vi "웹서버 온도 측정.vi"(6 "참조 번호 입력":T1 caption="client handle out", 7 "physical channels":tag caption="물리적 채널", 8 "error in":errorcluster caption="에러 입력", 9 "thermocouple type":i32(ring)=10072 caption="열전쌍 타입" items=["J"=10072, "K"=10073, "N"=10077, "R"=10082, "S"=10085, "T"=10086, "B"=10047, "E"=10055]) -> (0 "F포맷 문자열":string[](array[string]), 1 "error out":errorcluster, 2 "숫자형":i32, 3 "참조 번호 출력":T1 caption="client handle out", 4 "headers 3":string caption="연결확인 메세지 출력", 5 "온도값":string)   [LabVIEW 2019]
uses:
  <vilib>/httpClient/ClientHandle.ctl
  <vilib>/Analysis/baseanly.llb/Mean (DBL).vi
  <vilib>/DAQmx/read.llb/DAQmx Read (Analog 2D DBL NChan NSamp).vi
  <vilib>/DAQmx/create/channels.llb/DAQmx Create Channel (AI-Temperature-Thermocouple).vi
  <vilib>/DAQmx/configure/timing.llb/DAQmx Timing (Sample Clock).vi
  <vilib>/httpClient/PUTBuffer.vi
  <vilib>/DAQmx/miscellaneous.llb/DAQmx Fill In Error Info.vi
  <vilib>/Analysis/NI_AALBase.lvlib
  <vilib>/httpClient/LabVIEWHTTPClient.lvlib
panel:
  out "data":dbl[][](array[numeric]) caption="데이터" format="%0.2f"
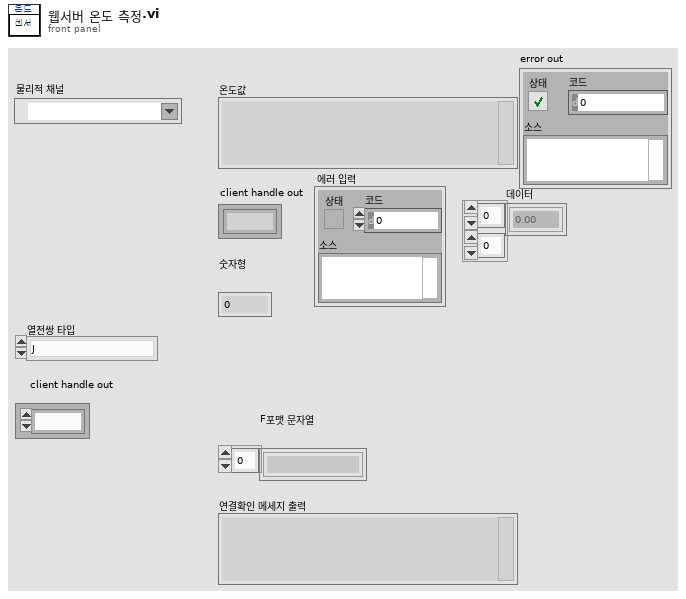
[diagram p1: front panel]
types:
  T1 = typedef "LabVIEWHTTPClient.lvlib/ClientHandle.ctl" = refnum<k1>
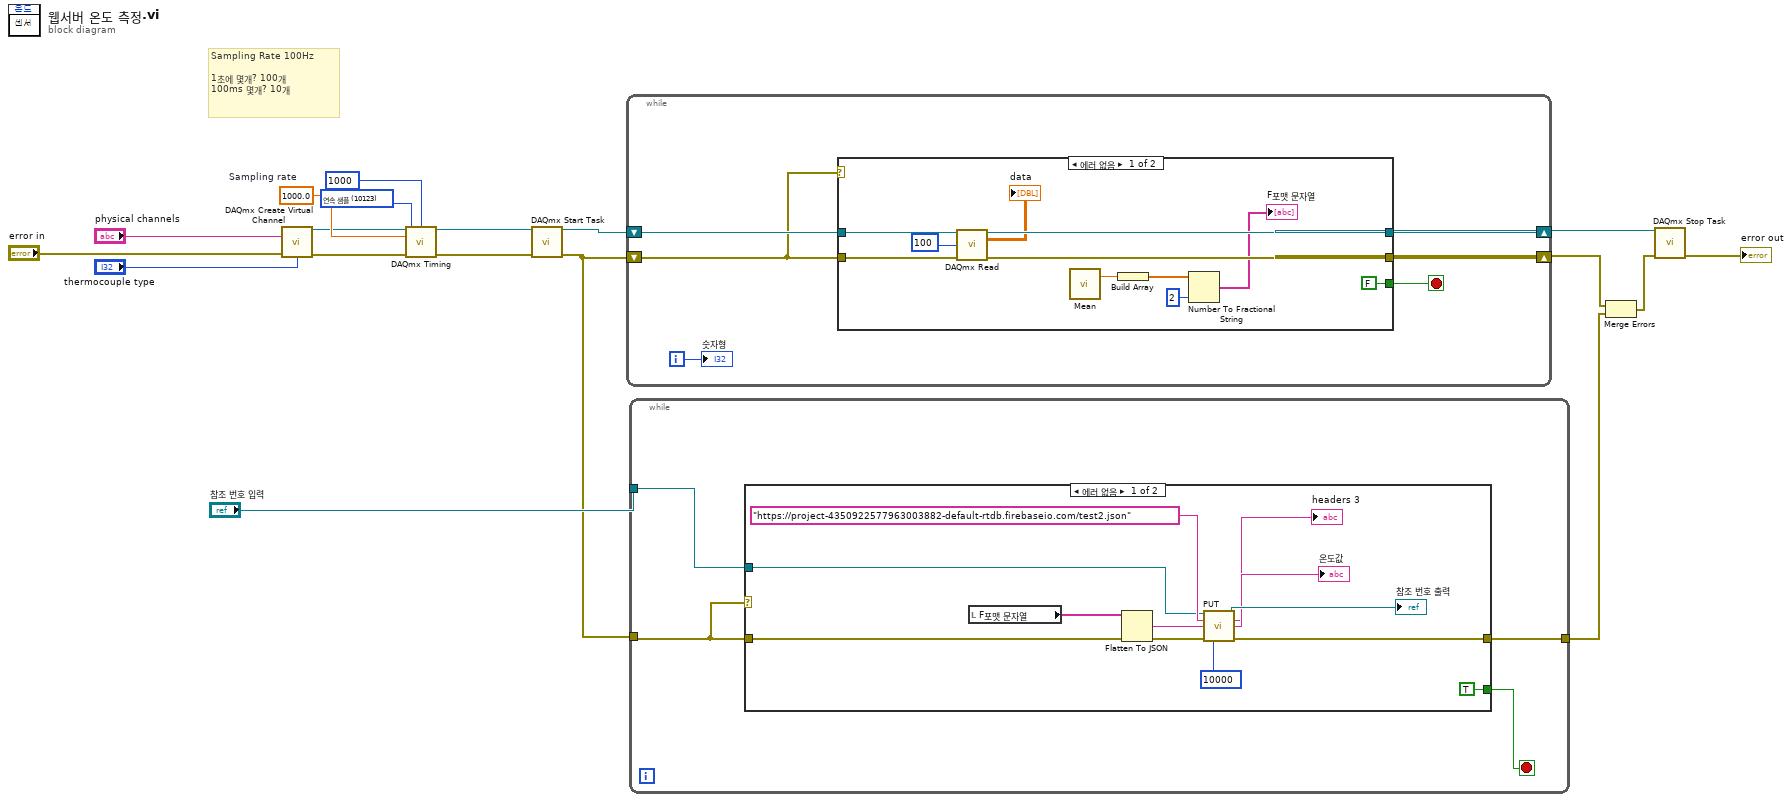
[diagram p0: block diagram]
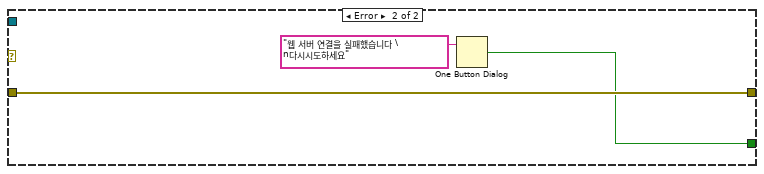
[diagram p2: hidden frame]
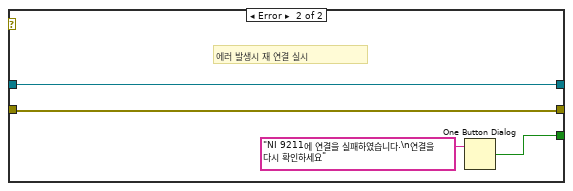
[diagram p3: hidden frame]
diagram:
  w9 = 1000.0  # Sampling rate
  w10 = 10123 items=["유한 샘플"=10178, "연속 샘플"=10123, "하드웨어 타이밍에 의한 단일 포인트"=12522] ("sample mode")
  # "Sampling Rate 100Hz\n\n1초에 몇개? 100개\n100ms 몇개? 10개"
  n1 = call-poly <vilib>:"DAQmx Create Virtual Channel.vi"("physical channels"="physical channels", "error in"="error in", "thermocouple type"="thermocouple type") -> ("task out"=w4:refnum<k21>, "error out"=w6:errorcluster)  [unwired: 11 in]
  n2 = call-poly <vilib>:"DAQmx Timing.vi"("task/channels in"=w4, "sample mode"=w10, "samples per channel"=1000, "rate"=w9, "error in"=w6) -> ("task out"=w5:refnum<k21>, "error out"=w7:errorcluster)  [unwired: 9 in]
  n3 = call <vilib>:"DAQmx Start Task.vi"("task/channels in"=w5, "error in"=w7) -> ("task out"=w12:refnum<k21>, "error out"=w13:errorcluster)  [unwired: 12 in]
  n4 = while {
    shift-right: [w23] -> w11
    shift-left: w12 -> [w24]
    shift-right: [w22] -> w3
    shift-left: w13 -> [w20]
    i -> [w21]
    stop <- w19 stop-if-true
    n5 = case shown="에러 없음" w20 {
      tunnel: w24 -> [w35 w39]
      tunnel: w20 -> [w34 w38]
      tunnel: [w33 w39] -> w23
      tunnel: [w32 w38] -> w22
      tunnel: [FALSE ("true") w36] -> w19
      frame No Error {
        n6 = call-poly <vilib>:"DAQmx Read.vi"("task/channels in"=w35, "number of samples per channel"=100, "error in"=w34) -> ("task out"=w33:refnum<k21>, "data"=→"data":dbl[][], "error out"=w32:errorcluster)  [unwired: 10 in]
        n7 = call-poly <vilib>:"Mean.vi"() -> ("mean"=w28:dbl)  [unwired: 1 in, 1 out]
        n8 = Build Array(w28) -> (w30:dbl[])
        n9 = Number To Fractional String(number=w30, precision (6)=i16 2 ("정밀도(6)")) -> (F-format string=→"F포맷 문자열":string[])  [unwired: 2 in]
      }
      frame Error {
        # "에러 발생시 재 연결 실시"
        n10 = One Button Dialog(message="NI 9211에 연결을 실패하였습니다.\n연결을 다시 확인하세요" ("메시지")) -> (true=w36:bool)  [unwired: 1 in]
      }
    }
    "숫자형" <- w21
  }
  n11 = while {
    tunnel: w13 -> [w41]
    tunnel: "참조 번호 입력" -> [w43]
    tunnel: [w42] -> w2
    stop <- w40 stop-if-true
    n12 = case shown="에러 없음" w41 {
      tunnel: w41 -> [w48 w57]
      tunnel: w43 -> [w47 _]
      tunnel: [w46 w57] -> w42
      tunnel: [TRUE ("true") w56] -> w40
      frame No Error {
        n13 = local read "F포맷 문자열"() -> (w45:string[])
        n14 = Flatten To JSON(anything=w45, error in (no error)=w48) -> (JSON string=w52:string, 11:w51:errorcluster)  [unwired: 1 in]
        n15 = call-poly <vilib>:"PUT.vi"("client handle"=w47, "url"="https://project-4350922577963003882-default-rtdb.firebaseio.com/test2.json", "buffer"=w52, "error in (no error)"=w51, "timeout (10000)"=10000) -> ("client handle out"=→"참조 번호 출력":T1, "headers"=→"headers 3":string, "body"=→"온도값":string, "error out"=w46:errorcluster)  [unwired: 7 in]
      }
      frame Error {
        n16 = One Button Dialog(message="웹 서버 연결을 실패했습니다 \n다시시도하세요" ("메시지")) -> (true=w56:bool)  [unwired: 1 in]
      }
    }
  }
  n17 = Merge Errors(w3, w2) -> (w1:errorcluster)
  n18 = call <vilib>:"DAQmx Stop Task.vi"("task/channels in"=w11, "error in"=w1) -> ("error out"=→"error out":errorcluster)  [unwired: 12 in, 1 out]
